vi "robot main3.vi"() -> ()   [LabVIEW 2014]
doc: "Tank Drive Example\n\nThis example shows how to implement tank drive and uses two joysticks for input.\n\nThis example expects a USB cable connected from your development PC to the Type B USB Jack (next to the power input) on the roboRIO.\n\nThis example requires the Driver Station to be running with Teleoperated Enabled."
uses:
  <vilib>/Rock Robotics/SystemInterfaces/DIO/FPGA_DIOPWMChannel.ctl
  <vilib>/Rock Robotics/WPI/Joystick/WPI_JoystickDeviceEnum.ctl
  <vilib>/Rock Robotics/WPI/Solenoid/WPI_SolenoidChannel.ctl
  <vilib>/Rock Robotics/WPI/Solenoid/WPI_SolenoidValue.ctl
  <vilib>/Rock Robotics/WPI/RobotDrive/WPI_RobotDriveOpen2MotorWithTalon.vi
  <vilib>/Rock Robotics/WPI/RobotDrive/WPI_RobotDriveOpen4MotorWithTalon.vi
  <vilib>/Rock Robotics/WPI/Solenoid/WPI_SolenoidOpenSingle.vi
  <vilib>/Rock Robotics/WPI/Solenoid/WPI_SolenoidSetEnum.vi
panel:
  in  "stop 2":bool
  in  "Value to Write":bool
  in  "stop":bool
  # "Set these inputs before running."
  # "This example requires the Driver Station to be running with Teleoperated Enabled."
  # "PWM cables"
  # "This shows wiring for Talon speed controllers.  The wiring is similar for Victor and Jaguar controllers.  If you change the controller type, you must also select the appropriate instance of the Motor Open VI on the diagram."
  # "Power\nTerminals"
  # "Motor\nTerminals"
  # "+"
  # "+"
  # "M"
  # "B"
  # "Power\nTerminals"
  # "Motor\nTerminals"
  # "+"
  # "+"
  # "M"
  # "B"
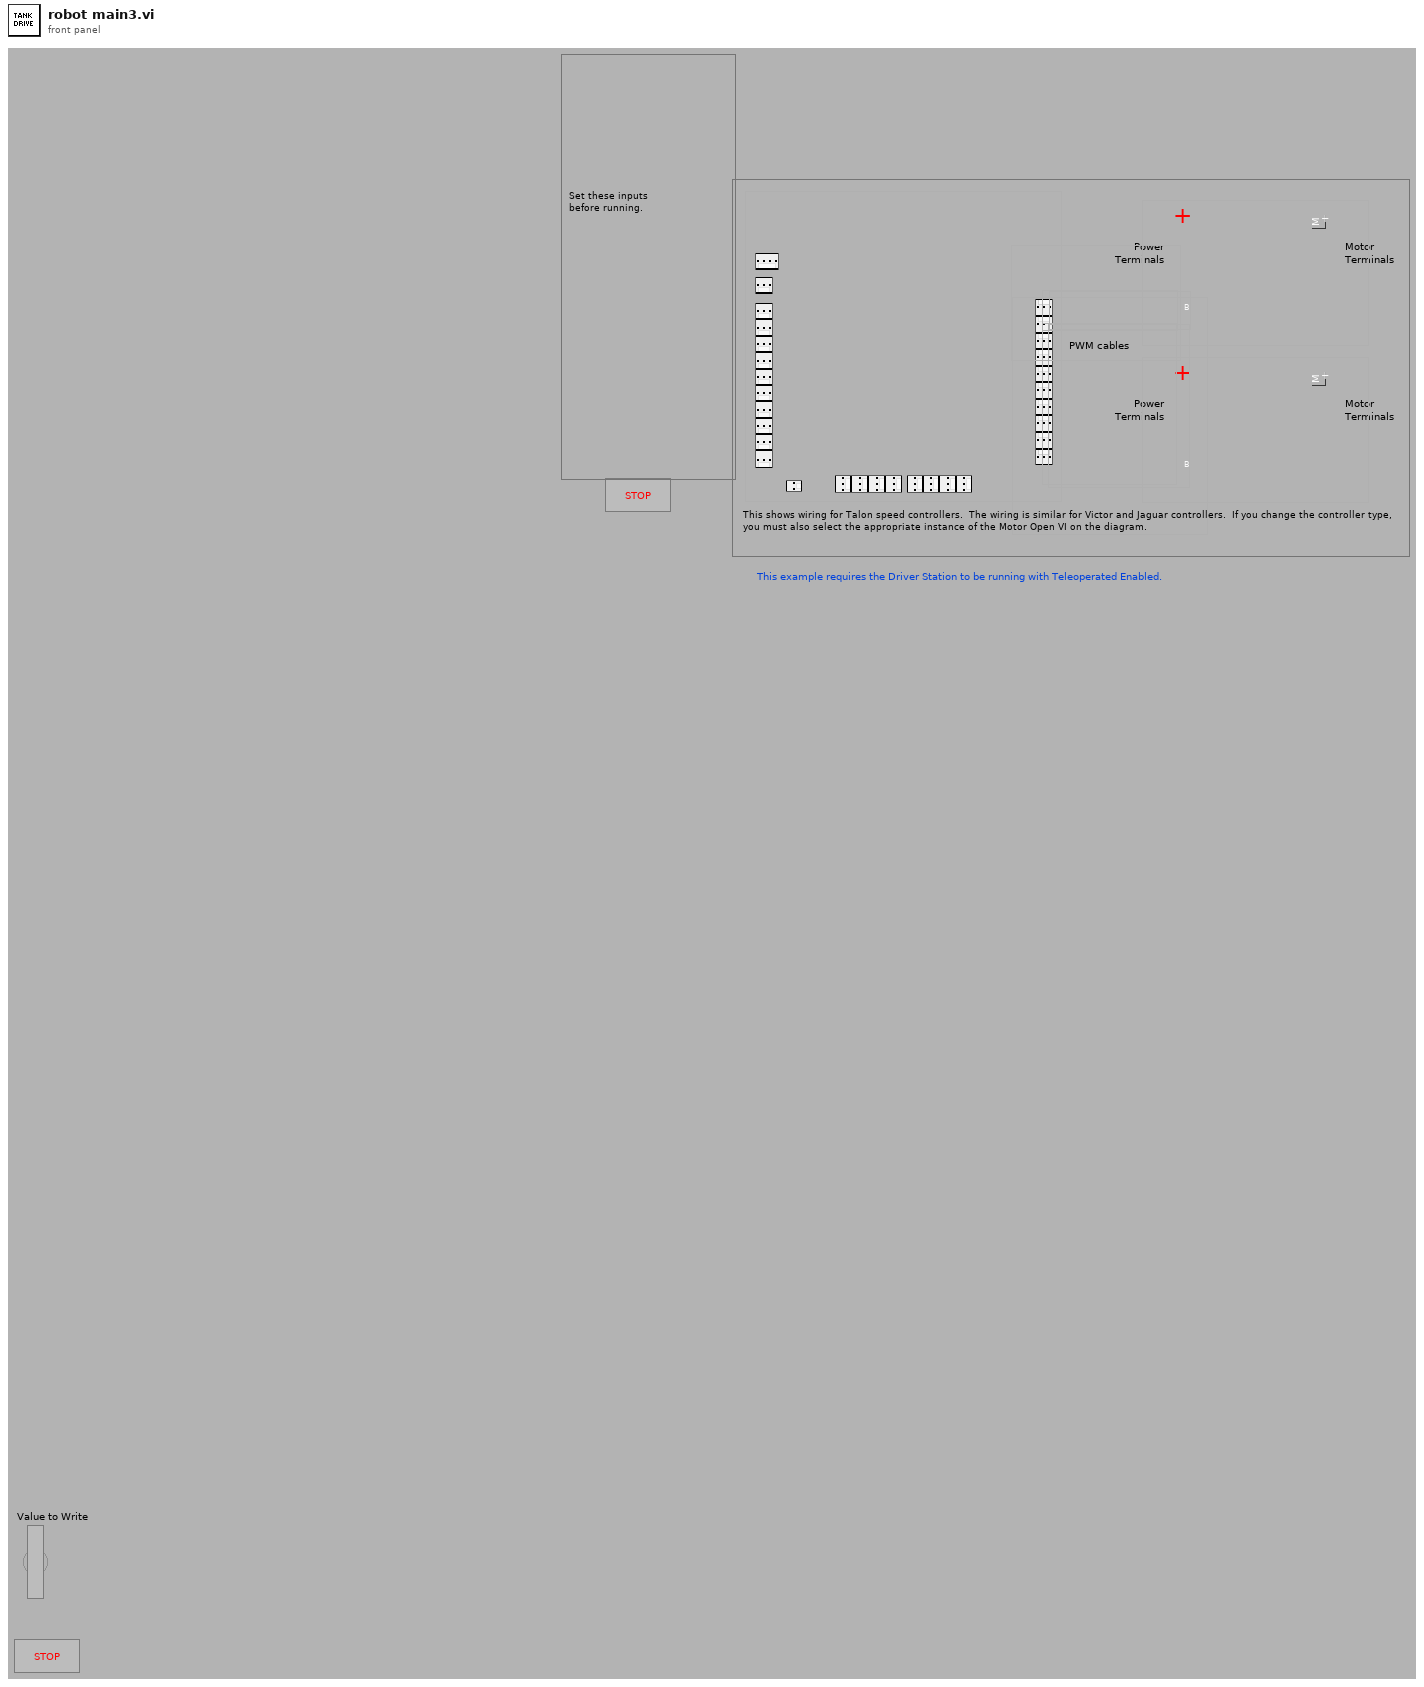
[diagram p1: front panel]
types:
  T1 = typedef "WPI_SolenoidChannel.ctl" = enum8{"Solenoid 0", "Solenoid 1", "Solenoid 2", "Solenoid 3", "Solenoid 4", "Solenoid 5", "Solenoid 6", "Solenoid 7", "Invalid"}
  T2 = typedef "WPI_JoystickDeviceEnum.ctl" = enum16{"USB 0", "USB 1", "USB 2", "USB 3", "USB 4", "USB 5"}
  T3 = typedef "FPGA_DIOPWMChannel.ctl" = enum8{"PWM 0", "PWM 1", "PWM 2", "PWM 3", "PWM 4", "PWM 5", "PWM 6", "PWM 7", "PWM 8", "PWM 9", "PWM MXP 0", "PWM MXP 1", "PWM MXP 2", "PWM MXP 3", "PWM MXP 4", "PWM MXP 5", "PWM MXP 6", "PWM MXP 7", "PWM MXP 8", "PWM MXP 9", "Invalid"}
  T4 = typedef "WPI_RobotDriveDevRef.ctl" = cluster{"DevStatus":errorcluster, "Motors[]":T5[], "Square Inputs":bool, "Max Output":dbl}
  T5 = typedef "WPI_MotorControlDeviceRef.ctl" = cluster{"DeviceStatus":errorcluster, "Type":T6, "PWM":cluster{"Controller":T7, "PWM Channel":T3, "DeadBand":T8}, "CAN":cluster{"Device Number":u8, "Control Mode":T9, "Semaphore":T10, "Max Vout":dbl, "TalonSRX Control Mode":T11}, "Invert":bool, "TransformRef":T12, "InvTransformRef":T12}
  T6 = typedef "WPI_MotorControlType.ctl" = enum16{"PWM", "CAN", "CANTalonSRX"}
  T7 = typedef "FPGA_TypedefDigitalModule.ctl" = enum16{"Controller 1"}
  T8 = typedef "WPI_PWMDeadband.ctl" = cluster{"Name":string, "maxPositivePwm":i32, "minPositivePwm":i32, "centerPwm":i32, "maxNegativePwm":i32, "minNegativePwm":i32, "angularRange":u16}
  T9 = typedef "WPI_CANJaguar_ControlMode.ctl" = enum8{"Percent VBus", "Current", "Speed", "Position", "Voltage"}
  T10 = typedef "Semaphore RefNum" = refnum<k1>
  T11 = typedef "WPI_CANTalonSRX_APIControlMode.ctl" = enum8{"Percent VBus", "Speed", "Position", "Slave", "Unchanged / Invalid"}
  T12 = typedef "WPI_PWMTransform_ConPane.ctl" = refnum<vi>
  T13 = typedef "WPI_SolenoidDevRef.ctl" = cluster{"DevStatus":errorcluster, "Pneumatics Control Module":u8, "Forward Solenoid Channel":T1, "Reverse Solenoid Channel":T1}
  T14 = typedef "WPI_JoystickDevRef.ctl" = cluster{"Device":T2}
  T15 = typedef "WPI_SolenoidValue.ctl" = enum16{"Off", "On", "Forward", "Reverse"}
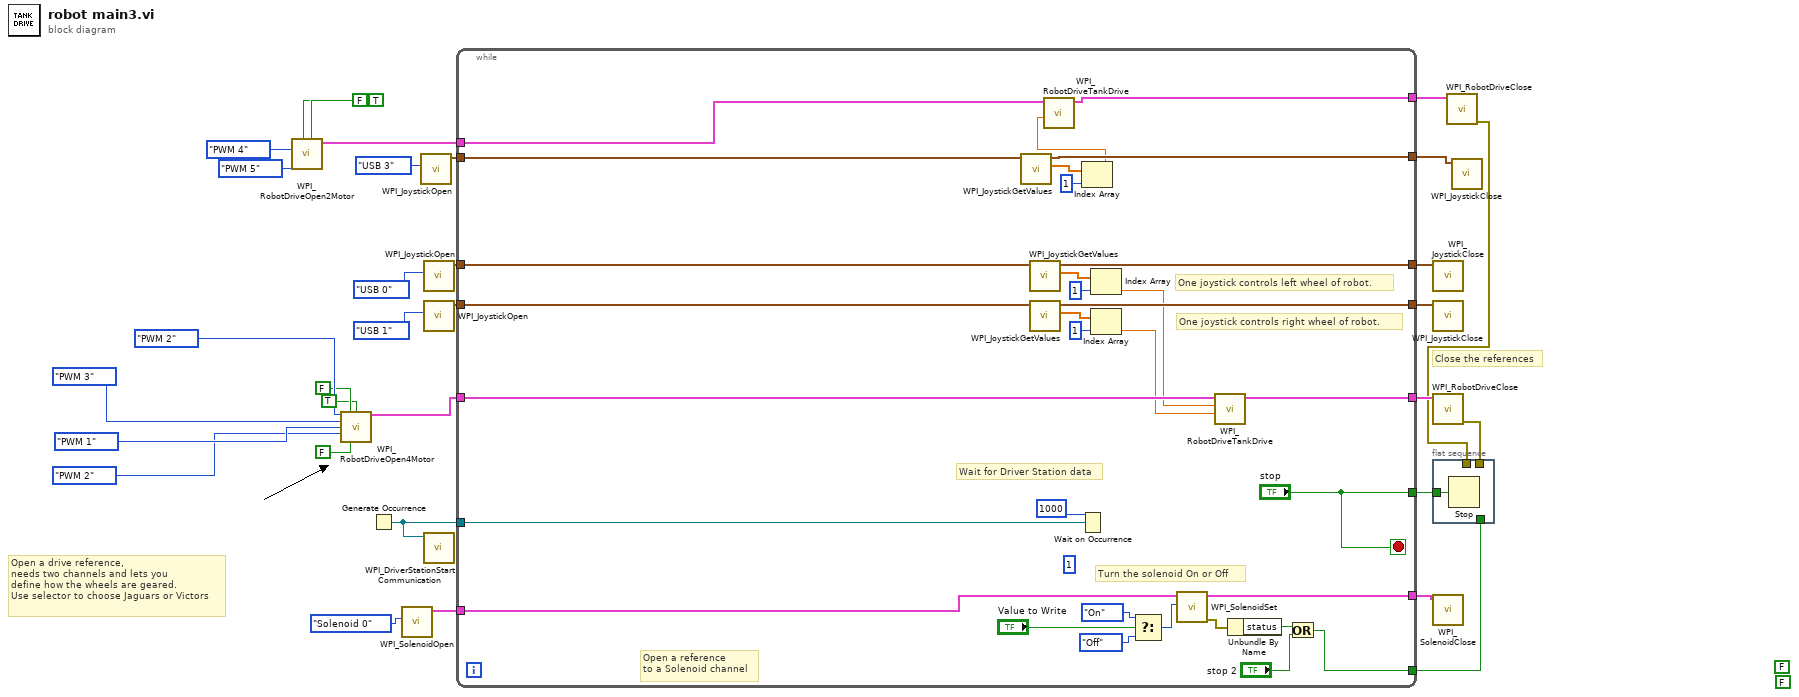
[diagram p0: block diagram]
diagram:
  (unwired) FALSE ("Right Motor Inverted")
  (unwired) FALSE ("Left Motor Inverted")
  # "Close the references"
  # "Open a drive reference,\nneeds two channels and lets you\ndefine how the wheels are geared.\nUse selector to choose Jaguars or Victors"
  n1 = call-poly <vilib>:"WPI_RobotDriveOpen2Motor.vi"("Right Motor Inverted"=TRUE, "Left Motor Inverted"=FALSE, "Right Motor"=FPGA_DIOPWMChannel."PWM 4", "Left Motor"=FPGA_DIOPWMChannel."PWM 5") -> ("RobotDriveDevRef"=w4:T4)  [unwired: 6 in, 1 out]
  n2 = call-poly <vilib>:"WPI_RobotDriveOpen4Motor.vi"("Rear Left Motor"=FPGA_DIOPWMChannel."PWM 2" ("Left Motor (PWM channel)"), "Rear Left Motor Inverted"=FALSE, "Rear Right Motor Inverted"=TRUE, "Rear Right Motor"=FPGA_DIOPWMChannel."PWM 3" ("Right Motor (PWM channel)"), "Front Left Motor"=FPGA_DIOPWMChannel."PWM 1", "Front Right Motor"=FPGA_DIOPWMChannel."PWM 2", "Front Left Motor Inverted"=FALSE) -> ("RobotDriveDevRef"=w20:T4)  [unwired: 7 in, 1 out]
  n3 = Generate Occurrence() -> (w31:refnum<k4>)
  n4 = call-poly <vilib>:"WPI_SolenoidOpen.vi"("Solenoid Channel"=WPI_SolenoidChannel."Solenoid 0") -> ("SolenoidDevRef"=w13:T13)  [unwired: 2 in, 8 out]
  n5 = call <vilib>:"WPI_JoystickOpen.vi"("JoystickDevice"=WPI_JoystickDeviceEnum."USB 3") -> ("JoystickDevRef"=w6:T14)  [unwired: 10 out]
  n6 = call <vilib>:"WPI_JoystickOpen.vi"("JoystickDevice"=WPI_JoystickDeviceEnum."USB 0" ("LeftStick")) -> ("JoystickDevRef"=w27:T14)  [unwired: 10 out]
  n7 = call <vilib>:"WPI_JoystickOpen.vi"("JoystickDevice"=WPI_JoystickDeviceEnum."USB 1" ("RightStick")) -> ("JoystickDevRef"=w28:T14)  [unwired: 10 out]
  n8 = call <vilib>:"WPI_DriverStationStart Communication.vi"("occurrence"=w31) -> ()  [unwired: 1 in, 10 out]
  n9 = while {
    tunnel: w20 -> [w59]
    tunnel: [w60] -> w32
    tunnel: w31 -> [w64]
    tunnel: ["stop"] -> w24
    tunnel: w28 -> [w62]
    tunnel: w27 -> [w61]
    tunnel: [w57] -> w26
    tunnel: [w56] -> w25
    tunnel: w13 -> [w43]
    tunnel: [w42] -> w12
    tunnel: [w40] -> w11
    tunnel: [w38] -> w7
    tunnel: w6 -> [w37]
    tunnel: w4 -> [w36]
    tunnel: [w35] -> w3
    stop <- "stop" stop-if-true
    (unwired) 1 ("index")
    # "Open a reference \nto a Solenoid channel"
    # "Turn the solenoid On or Off"
    # "Wait for Driver Station data"
    # "One joystick controls right wheel of robot."
    # "One joystick controls left wheel of robot."
    n10 = call <vilib>:"WPI_JoystickGetValues.vi"("JoystickDevRef"=w37) -> ("Axes"=w39:dbl[], "JoystickDevRef"=w38:T14)  [unwired: 6 in, 3 out]
    n11 = call <vilib>:"WPI_JoystickGetValues.vi"("JoystickDevRef"=w61) -> ("Axes"=w58:dbl[], "JoystickDevRef"=w57:T14)  [unwired: 6 in, 3 out]
    n12 = call <vilib>:"WPI_JoystickGetValues.vi"("JoystickDevRef"=w62) -> ("Axes"=w53:dbl[], "JoystickDevRef"=w56:T14)  [unwired: 6 in, 3 out]
    n13 = Wait on Occurrence(2:w64, 3:1000 ("ms timeout (-1)")) -> ()  [unwired: 2 out]
    n14 = Index Array(array=w39, index=1) -> (element=w33:dbl)
    n15 = call <vilib>:"WPI_RobotDriveTankDrive.vi"("Right axis value"=w33, "RobotDriveDevRef"=w36) -> ("RobotDriveDevRef"=w35:T4)  [unwired: 7 in, 2 out]
    n16 = Index Array(array=w58, index=1) -> (element=w52:dbl)
    n17 = Index Array(array=w53, index=1) -> (element=w51:dbl)
    n18 = Select(t=WPI_SolenoidValue."On" ("Value"), s="Value to Write", f=WPI_SolenoidValue."Off" ("Value")) -> (s? t:f=w44:T15)
    n19 = call-poly <vilib>:"WPI_SolenoidSet.vi"("Value"=w44, "SolenoidDevRef"=w43) -> ("error out"=w50:errorcluster, "SolenoidDevRef"=w42:T13)  [unwired: 1 in, 7 out]
    n20 = call <vilib>:"WPI_RobotDriveTankDrive.vi"("Right axis value"=w51, "Left axis value"=w52, "RobotDriveDevRef"=w59) -> ("RobotDriveDevRef"=w60:T4)  [unwired: 1 in, 7 out]
    n21 = Unbundle By Name(w50) -> ("status"=w49:bool)
    n22 = Or(x=w49, y="stop 2") -> (x .or. y?=w40:bool)
  }
  n23 = call <vilib>:"WPI_JoystickClose.vi"("JoystickDevRef"=w26) -> ()  [unwired: 11 out]
  n24 = call <vilib>:"WPI_JoystickClose.vi"("JoystickDevRef"=w25) -> ()  [unwired: 11 out]
  n25 = call <vilib>:"WPI_RobotDriveClose.vi"("RobotDriveDevRef"=w32) -> ("error out"=w23:errorcluster)  [unwired: 1 in, 9 out]
  n26 = flat-sequence {
    tunnel: w24 -> [w65]
    tunnel: w23 -> [_]
    tunnel: w11 -> [_]
    tunnel: w5 -> [_]
    frame #0 {
      n27 = Stop(stop? (T)=w65) -> ()
    }
  }
  n28 = call <vilib>:"WPI_SolenoidClose.vi"("SolenoidDevRef"=w12) -> ()  [unwired: 10 in, 1 out]
  n29 = call <vilib>:"WPI_RobotDriveClose.vi"("RobotDriveDevRef"=w3) -> ("error out"=w5:errorcluster)  [unwired: 10 in]
  n30 = call <vilib>:"WPI_JoystickClose.vi"("JoystickDevRef"=w7) -> ()  [unwired: 11 in]
